vi "SubVI_Resize_RGB_Array #.vi"(7 "Magnification":i32 min=0 max=9 step=1, 8 "Error In":errorcluster, 11 "Image In":T1) -> (0 "Error Out":errorcluster, 1 "B":u8[][](array[numeric]), 2 "G":u8[][](array[numeric]), 3 "R":u8[][](array[numeric]))   [LabVIEW 2013]
uses:
  <vilib>/vision/Image Controls.llb/IMAQ Image.ctl
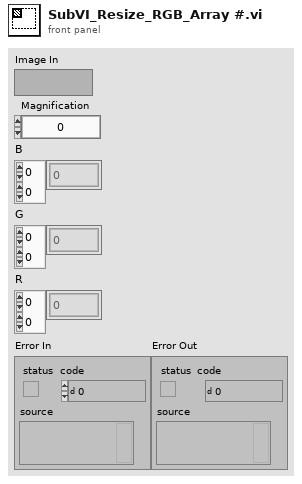
[diagram p1: front panel]
types:
  T1 = typedef "IMAQ Image.ctl" = refnum<image>
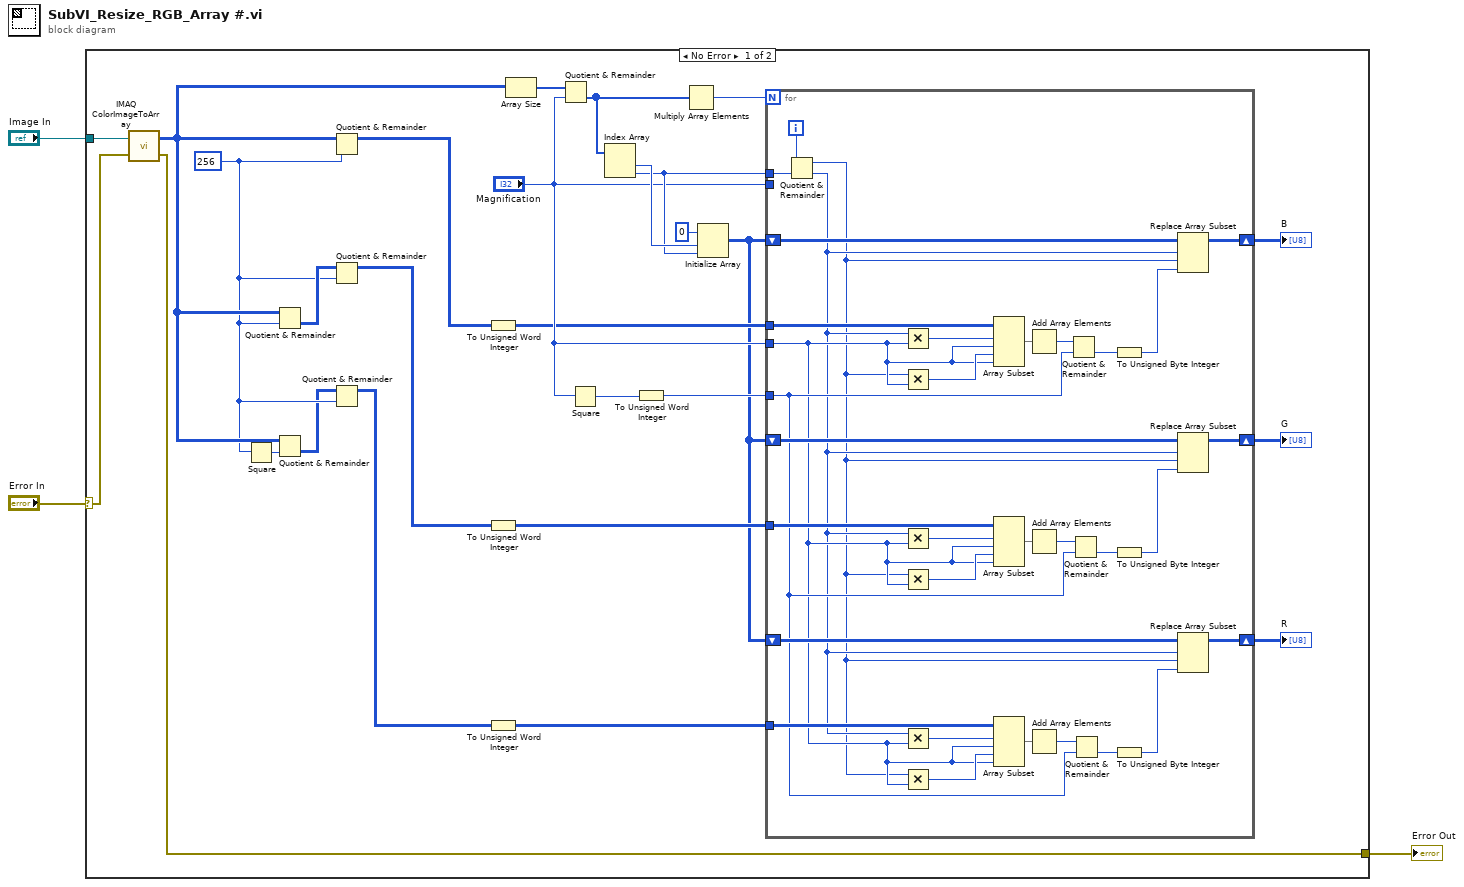
[diagram p0: block diagram]
diagram:
  n1 = case shown="No Error" "Error In" {
    selector: "Error In" -> [w5 w64]
    tunnel: "Image In" -> [w7 _]
    tunnel: [w6 w64] -> w2
    frame No Error {
      w11 = u32 256 ("y")
      n2 = call "IMAQ ColorImageToArray"("Image"=w7, "error in (no error)"=w5) -> ("Image Pixels (U32)"=w12:u32[][], "error out"=w6:errorcluster)  [unwired: 2 in, 1 out]
      n3 = Square(x=w11) -> (x^2=w30:u32)
      n4 = Quotient & Remainder(x=w12, y=w11) -> (floor(x/y)=w29:u32[][])  [unwired: 1 out]
      n5 = Quotient & Remainder(x=w12, y=w30) -> (floor(x/y)=w4:u32[][])  [unwired: 1 out]
      n6 = Quotient & Remainder(x=w12, y=w11) -> (x-y*floor(x/y)=w15:u32[][])  [unwired: 1 out]
      n7 = Quotient & Remainder(x=w29, y=w11) -> (x-y*floor(x/y)=w14:u32[][])  [unwired: 1 out]
      n8 = Quotient & Remainder(x=w4, y=w11) -> (x-y*floor(x/y)=w13:u32[][])  [unwired: 1 out]
      n9 = To Unsigned Word Integer(number=w15) -> (unsigned 16bit integer=w21:u16[][])
      n10 = To Unsigned Word Integer(number=w14) -> (unsigned 16bit integer=w18:u16[][])
      n11 = To Unsigned Word Integer(number=w13) -> (unsigned 16bit integer=w16:u16[][])
      n12 = Array Size(array=w12) -> (size(s)=w28:i32[])
      n13 = Quotient & Remainder(x=w28, y="Magnification") -> (floor(x/y)=w27:i32[])  [unwired: 1 out]
      n14 = Square(x="Magnification") -> (x^2=w20:i32)
      n15 = Index Array(array=w27) -> (element #1=w24:i32, element #2=w23:i32)  [unwired: 2 in]
      n16 = To Unsigned Word Integer(number=w20) -> (unsigned 16bit integer=w19:u16)
      n17 = Multiply Array Elements(1:w27) -> (0:w26:i32)
      n18 = Initialize Array(u8 0 ("element"), w24, w23) -> (w17:u8[][])
      n19 = for {
        N: w26 -> [_]
        tunnel: w21 -> [w58]
        tunnel: w23 -> [w63]
        shift-right: [w61] -> w10
        shift-left: w17 -> [w60]
        tunnel: "Magnification" -> [_]
        tunnel: "Magnification" -> [w33]
        tunnel: w19 -> [w34]
        shift-right: [w45] -> w9
        shift-left: w17 -> [w46]
        tunnel: w18 -> [w44]
        shift-right: [w42] -> w8
        shift-left: w17 -> [w41]
        tunnel: w16 -> [w43]
        i -> [w62]
        n20 = Quotient & Remainder(x=w62, y=w63) -> (x-y*floor(x/y)=w31:i32, floor(x/y)=w32:i32)
        n21 = Multiply(x=w32, y=w33) -> (x*y=w57:i32)
        n22 = Multiply(x=w31, y=w33) -> (x*y=w56:i32)
        n23 = Multiply(x=w32, y=w33) -> (x*y=w48:i32)
        n24 = Multiply(x=w31, y=w33) -> (x*y=w49:i32)
        n25 = Multiply(x=w32, y=w33) -> (x*y=w39:i32)
        n26 = Multiply(x=w31, y=w33) -> (x*y=w38:i32)
        n27 = Array Subset(array=w58, index (row)=w57, length (row)=w33, index (col)=w56, length (col)=w33) -> (w59:u16[][])
        n28 = Array Subset(array=w44, index (row)=w48, length (row)=w33, index (col)=w49, length (col)=w33) -> (w47:u16[][])
        n29 = Array Subset(array=w43, index (row)=w39, length (row)=w33, index (col)=w38, length (col)=w33) -> (w40:u16[][])
        n30 = Add Array Elements(numeric array=w59) -> (sum=w53:u16)
        n31 = Add Array Elements(numeric array=w47) -> (sum=w52:u16)
        n32 = Add Array Elements(numeric array=w40) -> (sum=w35:u16)
        n33 = Quotient & Remainder(x=w53, y=w34) -> (floor(x/y)=w55:u16)  [unwired: 1 out]
        n34 = Quotient & Remainder(x=w52, y=w34) -> (floor(x/y)=w50:u16)  [unwired: 1 out]
        n35 = Quotient & Remainder(x=w35, y=w34) -> (floor(x/y)=w37:u16)  [unwired: 1 out]
        n36 = To Unsigned Byte Integer(number=w55) -> (unsigned 8bit integer=w54:u8)
        n37 = To Unsigned Byte Integer(number=w50) -> (unsigned 8bit integer=w51:u8)
        n38 = To Unsigned Byte Integer(number=w37) -> (unsigned 8bit integer=w36:u8)
        n39 = Replace Array Subset(array=w60, new element=w54, index (row)=w32, index (col)=w31) -> (w61:u8[][])
        n40 = Replace Array Subset(array=w46, new element=w51, index (row)=w32, index (col)=w31) -> (w45:u8[][])
        n41 = Replace Array Subset(array=w41, new element=w36, index (row)=w32, index (col)=w31) -> (w42:u8[][])
      }
      "B" <- w10
      "G" <- w9
      "R" <- w8
    }
    frame Error {
    }
  }
  "Error Out" <- w2
